vi "Bertta_v09_92.vi"() -> ()   [LabVIEW 2015]
panel:
  out "element":bool
  out "Started:":string
  in  "SHUTDOWN":bool
  in  "MASTER CONTROL":bool
  in  "Tab Control":T1(tab)
  out "Output File":path caption="selected path"
  in  "Browse folder":path=path "" caption="start path"
  in  "Read Seq":bool
  in  "Save Seq":bool
  in  "Configuration file":path=path "C:/Users/shresplab/Desktop/BerttaConfiguration.lvm" caption="Filename"
  in  "OK Button 2":bool
  out "Boolean":bool
  in  "User (initials)":string
  in  "Project name":string
  in  "Description":string
  out "PUMP1":bool
  out "Target amount":dbl
  out "Scale weight":dbl
  out "Amount now":dbl
  out "Flow rate":dbl
  out "Time to target":dbl format="%<%H:%M:%S>t"
  out "Current step":dbl
  out "Target":dbl
  out "Amount now":dbl
  out "Amount now":dbl
  out "Target":dbl
  out "Current step":dbl
  out "Time to target":dbl format="%<%H:%M:%S>t"
  out "Flow rate":dbl
  out "Amount now":dbl
  out "Scale weight":dbl
  out "Target amount":dbl
  out "PUMP2":bool
  out "Sensor OK 6":bool
  out "Sensor OK 5":bool
  out "Sensor OK 4":bool
  out "Sensor OK 3":bool
  in  "OK Button":bool
  in  "Add comment":string
  out "PUMP3":bool
  out "Target amount":dbl
  out "Scale weight":dbl
  out "Amount now":dbl
  out "Flow rate":dbl
  out "Time to target":dbl format="%<%H:%M:%S>t"
  out "Current step":dbl
  out "Target":dbl
  out "Amount now":dbl
  out "Tr":dbl
  out "Tj in":dbl
  out "Tj out":dbl
  out "T set":dbl
  out "Current step":i32
  out "RPM":dbl
  out "Torque 2":dbl
  out "Waveform Chart 5":dynamicdata(graph)
  out "Waveform Chart 6":dynamicdata(graph)
  out "Waveform Chart 7":dynamicdata(graph)
  in  "Tab Control 2":T2(tab)
  out "Waveform Chart 3":dynamicdata(graph)
  out "Waveform Chart 8":dynamicdata(graph)
  out "Waveform Chart 11":dynamicdata(graph)
  out "Waveform Chart 13":dynamicdata(graph)
  out "Waveform Chart 9":dynamicdata(graph)
  out "Table":string[][](table)=[["14.8.2017 18.06.59", "0,000000", "417,670000", "-0,150000", "1,000000", "22,220000", "23,366837", "23,574959", "23,985852", "23,690000", "240,000000", "4,000000", "0,000000", "397,000000", "-397,000000", "1,000000"], ["14.8.2017 18.07.06", "0,000000", "417,640000", "-0,120000", "1,000000", "22,220000", "23,763115", "23,906257", "23,985694", "23,680000", "240,000000", "4,000000", "0,000000", "397,000000", "-397,000000", "1,000000"], ["14.8.2017 18.07.13", "0,000000", "417,640000", "-0,120000", "1,000000", "22,220000", "23,965922", "24,013440", "23,984906", "23,670000", "240,000000", "4,100000", "3,000000", "397,000000", "-397,000000", "1,000000"], ["14.8.2017 18.07.21", "0,000000", "417,640000", "-0,120000", "1,000000", "22,220000", "23,943860", "23,900110", "23,987113", "23,670000", "240,000000", "4,000000", "0,000000", "397,000000", "-397,000000", "1,000000"], ["14.8.2017 18.07.28", "0,000000", "417,640000", "-0,120000", "1,000000", "22,220000", "23,736328", "23,600018", "23,989004", "23,660000", "240,000000", "4,000000", "0,000000", "397,000000", "-397,000000", "1,000000"], ["14.8.2017 18.07.36", "0,000000", "417,640000", "-0,120000", "1,000000", "22,220000", "23,480910", "23,324538", "23,991053", "23,660000", "240,000000", "4,000000", "0,000000", "397,000000", "-397,000000", "1,000000"], ["14.8.2017 18.07.43", "0,000000", "417,640000", "-0,120000", "2,000000", "22,220000", "23,195579", "23,008270", "23,999093", "23,650000", "240,000000", "4,000000", "0,000000", "397,000000", "-397,000000", "1,000000"], ["14.8.2017 18.07.51", "0,000000", "417,650000", "-417,650000", "1,000000", "22,220000", "22,862541", "22,649021", "24,003979", "23,650000", "240,000000", "4,000000", "0,000000", "397,000000", "-397,000000", "2,000000"], ["14.8.2017 18.07.58", "0,000000", "417,640000", "0,010000", "1,000000", "22,220000", "22,541353", "22,354878", "24,005398", "23,650000", "240,000000", "4,000000", "0,000000", "397,000000", "-397,000000", "1,000000"], ["14.8.2017 18.08.06", "0,000000", "417,640000", "0,010000", "1,000000", "22,220000", "22,347931", "22,253738", "24,007605", "23,640000", "240,000000", "4,100000", "0,000000", "397,000000", "-397,000000", "1,000000"], ["14.8.2017 18.08.13", "0,000000", "417,640000", "0,010000", "1,000000", "22,220000", "22,329030", "22,302102", "24,006028", "23,640000", "240,000000", "4,000000", "0,000000", "395,820000", "-395,820000", "1,000000"], ["14.8.2017 18.08.20", "0,000000", "417,640000", "0,010000", "1,000000", "22,220000", "22,466849", "22,511320", "24,002403", "23,630000", "240,000000", "4,000000", "0,000000", "395,830000", "-0,010000", "1,000000"], ["14.8.2017 18.08.28", "0,000000", "417,640000", "0,010000", "1,000000", "22,220000", "22,707062", "22,835101", "24,000984", "23,620000", "240,000000", "4,000000", "0,000000", "395,830000", "-0,010000", "1,000000"], ["14.8.2017 18.08.35", "0,000000", "417,640000", "0,010000", "1,000000", "22,220000", "23,054104", "23,232979", "24,001299", "23,600000", "240,000000", "4,000000", "0,000000", "395,830000", "-0,010000", "1,000000"], ["14.8.2017 18.08.43", "0,000000", "417,640000", "0,010000", "1,000000", "22,220000", "23,412371", "23,522793", "24,002560", "23,590000", "240,000000", "4,000000", "0,000000", "395,820000", "0,000000", "1,000000"], ["14.8.2017 18.08.51", "0,000000", "417,640000", "0,010000", "1,000000", "22,220000", "23,596247", "23,656125", "24,003821", "23,580000", "240,000000", "4,000000", "0,000000", "395,820000", "0,000000", "1,000000"]]
  in  "?":bool
  in  "Time":dbl format="Time to target (min):                %#_g"
  out "Current temp":dbl format="Current temperature (S1):   %#_6g"
  in  "OK Button 3":bool
  in  "T ext / T ext 2":enum32{"Sensor 1", "Sensor 2"}(radio)
  out "Sensor OK":bool
  in  "T fail":dbl=20.0 format="Failsafe temperature:              %#_g"
  in  "Setpoint":dbl=20.0 format="Temperature target:                %#_6g"
  in  "Manual select":T3(radio)
  out "Waveform Chart":dynamicdata(graph)
  out "T external 2":dbl format="Current temperature (S2):    %#_g"
  in  "UPDATE TEMP":bool
  out "Led11 5":bool
  out "RPM":dbl format="%_4f"
  out "Led10 3":bool
  out "Led9 3":bool
  out "Led8 3":bool
  out "Led7 3":bool
  out "Led6 3":bool
  out "Led5 3":bool
  out "Led4 3":bool
  out "Led3 3":bool
  out "Led2 3":bool
  out "Led1 3":bool
  in  "PumpSeq 4":dbl[][](array[numeric])=[[1.0, 1.0, 0.0, 0.0, 0.0, 0.0, 0.0, 0.0, 0.0, 0.0], [2.0, 1.0, 0.0, 0.0, 0.0, 0.0, 0.0, 0.0, 0.0, 0.0], [3.0, 1.0, 0.0, 0.0, 0.0, 0.0, 0.0, 0.0, 0.0, 0.0], [0.0, 0.0, 0.0, 0.0, 0.0, 0.0, 0.0, 0.0, 0.0, 0.0], [0.0, 0.0, 0.0, 0.0, 0.0, 0.0, 0.0, 0.0, 0.0, 0.0], [0.0, 0.0, 0.0, 0.0, 0.0, 0.0, 0.0, 0.0, 0.0, 0.0], [0.0, 0.0, 0.0, 0.0, 0.0, 0.0, 0.0, 0.0, 0.0, 0.0], [0.0, 0.0, 0.0, 0.0, 0.0, 0.0, 0.0, 0.0, 0.0, 0.0], [0.0, 0.0, 0.0, 0.0, 0.0, 0.0, 0.0, 0.0, 0.0, 0.0], [0.0, 0.0, 0.0, 0.0, 0.0, 0.0, 0.0, 0.0, 0.0, 0.0]]
  in  "?":bool
  out "Flow rate (g/min)":dbl
  out "Scale reading":dbl
  out "Step amount now":dbl
  in  "Grams / min":dbl
  out "Waveform Chart 14":dynamicdata(graph)
  in  "?":bool
  out "Total amount now":dbl
  out "Led11 4":bool
  in  "Reset 5":bool
  out "Elapsed / step":i32
  out "Time to target":dbl format="%<%H:%M:%S>t"
  in  "OK Button 4":bool
  out "Led11":bool
  out "RPM":dbl format="%_4f"
  out "Led10":bool
  out "Led9":bool
  out "Led8":bool
  out "Led7":bool
  out "Led6":bool
  out "Led5":bool
  out "Led4":bool
  out "Led3":bool
  out "Led2":bool
  out "Led1":bool
  in  "PumpSeq 2":dbl[][](array[numeric])=[[1.0, 2.0, 0.0, 0.0, 0.0, 0.0, 0.0, 0.0, 0.0, 0.0], [2.0, 2.0, 0.0, 0.0, 0.0, 0.0, 0.0, 0.0, 0.0, 0.0], [3.0, 2.0, 0.0, 0.0, 0.0, 0.0, 0.0, 0.0, 0.0, 0.0], [0.0, 0.0, 0.0, 0.0, 0.0, 0.0, 0.0, 0.0, 0.0, 0.0], [0.0, 0.0, 0.0, 0.0, 0.0, 0.0, 0.0, 0.0, 0.0, 0.0], [0.0, 0.0, 0.0, 0.0, 0.0, 0.0, 0.0, 0.0, 0.0, 0.0], [0.0, 0.0, 0.0, 0.0, 0.0, 0.0, 0.0, 0.0, 0.0, 0.0], [0.0, 0.0, 0.0, 0.0, 0.0, 0.0, 0.0, 0.0, 0.0, 0.0], [0.0, 0.0, 0.0, 0.0, 0.0, 0.0, 0.0, 0.0, 0.0, 0.0], [0.0, 0.0, 0.0, 0.0, 0.0, 0.0, 0.0, 0.0, 0.0, 0.0]]
  in  "?":bool
  out "Flow rate (g/min)":dbl
  out "Scale reading":dbl
  out "Step amount now":dbl
  in  "Grams / min":dbl
  out "Waveform Chart 10":dynamicdata(graph)
  in  "?":bool
  out "Total amount now":dbl
  out "Led11":bool
  in  "Reset 3":bool
  out "Elapsed / step":i32
  out "Time to target":dbl format="%<%H:%M:%S>t"
  in  "OK Button 5":bool
  out "Led11 3":bool
  out "RPM":dbl format="%_4f"
  out "Led10 2":bool
  out "Led9 2":bool
  out "Led8 2":bool
  out "Led7 2":bool
  out "Led6 2":bool
  out "Led5 2":bool
  out "Led4 2":bool
  out "Led3 2":bool
  out "Led2 2":bool
  out "Led1 2":bool
  in  "PumpSeq 3":dbl[][](array[numeric])=[[1.0, 3.0, 0.0, 0.0, 0.0, 0.0, 0.0, 0.0, 0.0, 0.0], [2.0, 3.0, 0.0, 0.0, 0.0, 0.0, 0.0, 0.0, 0.0, 0.0], [3.0, 3.0, 0.0, 0.0, 0.0, 0.0, 0.0, 0.0, 0.0, 0.0], [0.0, 0.0, 0.0, 0.0, 0.0, 0.0, 0.0, 0.0, 0.0, 0.0], [0.0, 0.0, 0.0, 0.0, 0.0, 0.0, 0.0, 0.0, 0.0, 0.0], [0.0, 0.0, 0.0, 0.0, 0.0, 0.0, 0.0, 0.0, 0.0, 0.0], [0.0, 0.0, 0.0, 0.0, 0.0, 0.0, 0.0, 0.0, 0.0, 0.0], [0.0, 0.0, 0.0, 0.0, 0.0, 0.0, 0.0, 0.0, 0.0, 0.0], [0.0, 0.0, 0.0, 0.0, 0.0, 0.0, 0.0, 0.0, 0.0, 0.0], [0.0, 0.0, 0.0, 0.0, 0.0, 0.0, 0.0, 0.0, 0.0, 0.0]]
  in  "?":bool
  out "Flow rate (g/min)":dbl
  out "Scale reading":dbl
  out "Step amount now":dbl
  in  "Grams / min":dbl
  out "Waveform Chart 12":dynamicdata(graph)
  in  "?":bool
  out "Total amount now":dbl
  out "Led11 2":bool
  in  "Reset 4":bool
  out "Elapsed / step":i32
  out "Time to target":dbl format="%<%H:%M:%S>t"
  in  "OK Button 6":bool
  in  "Bypass select 2":enum32{"Remote", "Manual"}(radio)=enum."Manual"
  in  "Port":dbl=13.0
  out "RPM":dbl
  out "Torque":dbl
  in  "Set RPM":dbl(slide) scale=0.0..2000.0
  out "Waveform Chart 4":dynamicdata(graph)
  in  "OK Button 7":bool
  out "output array":dbl[](array[numeric])
  in  "dev1":i32=1
  in  "dev2":i32=2
  in  "dev3":i32=3
  in  "dev4":i32=4
  in  "dev5":i32=5
  in  "dev6":i32=5
  in  "dev8":i32
  in  "port1":i32=9
  in  "port2":i32=9
  in  "port3":i32=13
  in  "port4":i32=13
  in  "port5":i32=10
  in  "port6":i32=11
  in  "port7":i32=12
  in  "port8":i32
  in  "dev7":i32=5
  in  "Treshold (T/C)":dbl=0.5
  out "DAQ 9217 (PT100)":errorcluster
  out "Config File":dbl[][](array[numeric])
  # "Temperature sensor:"
  # "Manual control:"
  # "PUMP & SCALE 1"
  # "STEP"
  # "TOTAL"
  # "PUMP & SCALE 2"
  # "STEP"
  # "TOTAL"
  # "PUMP & SCALE 3"
  # "STEP"
  # "TOTAL"
  # "Temperature control parameter"
  # "Secondary temperature sensor"
  # "Grams    /   min"
  # "End of sequence"
  # "Manual control"
  # "Grams    /   min"
  # "End of sequence"
  # "Manual control"
  # "Grams    /   min"
  # "End of sequence"
  # "Manual control"
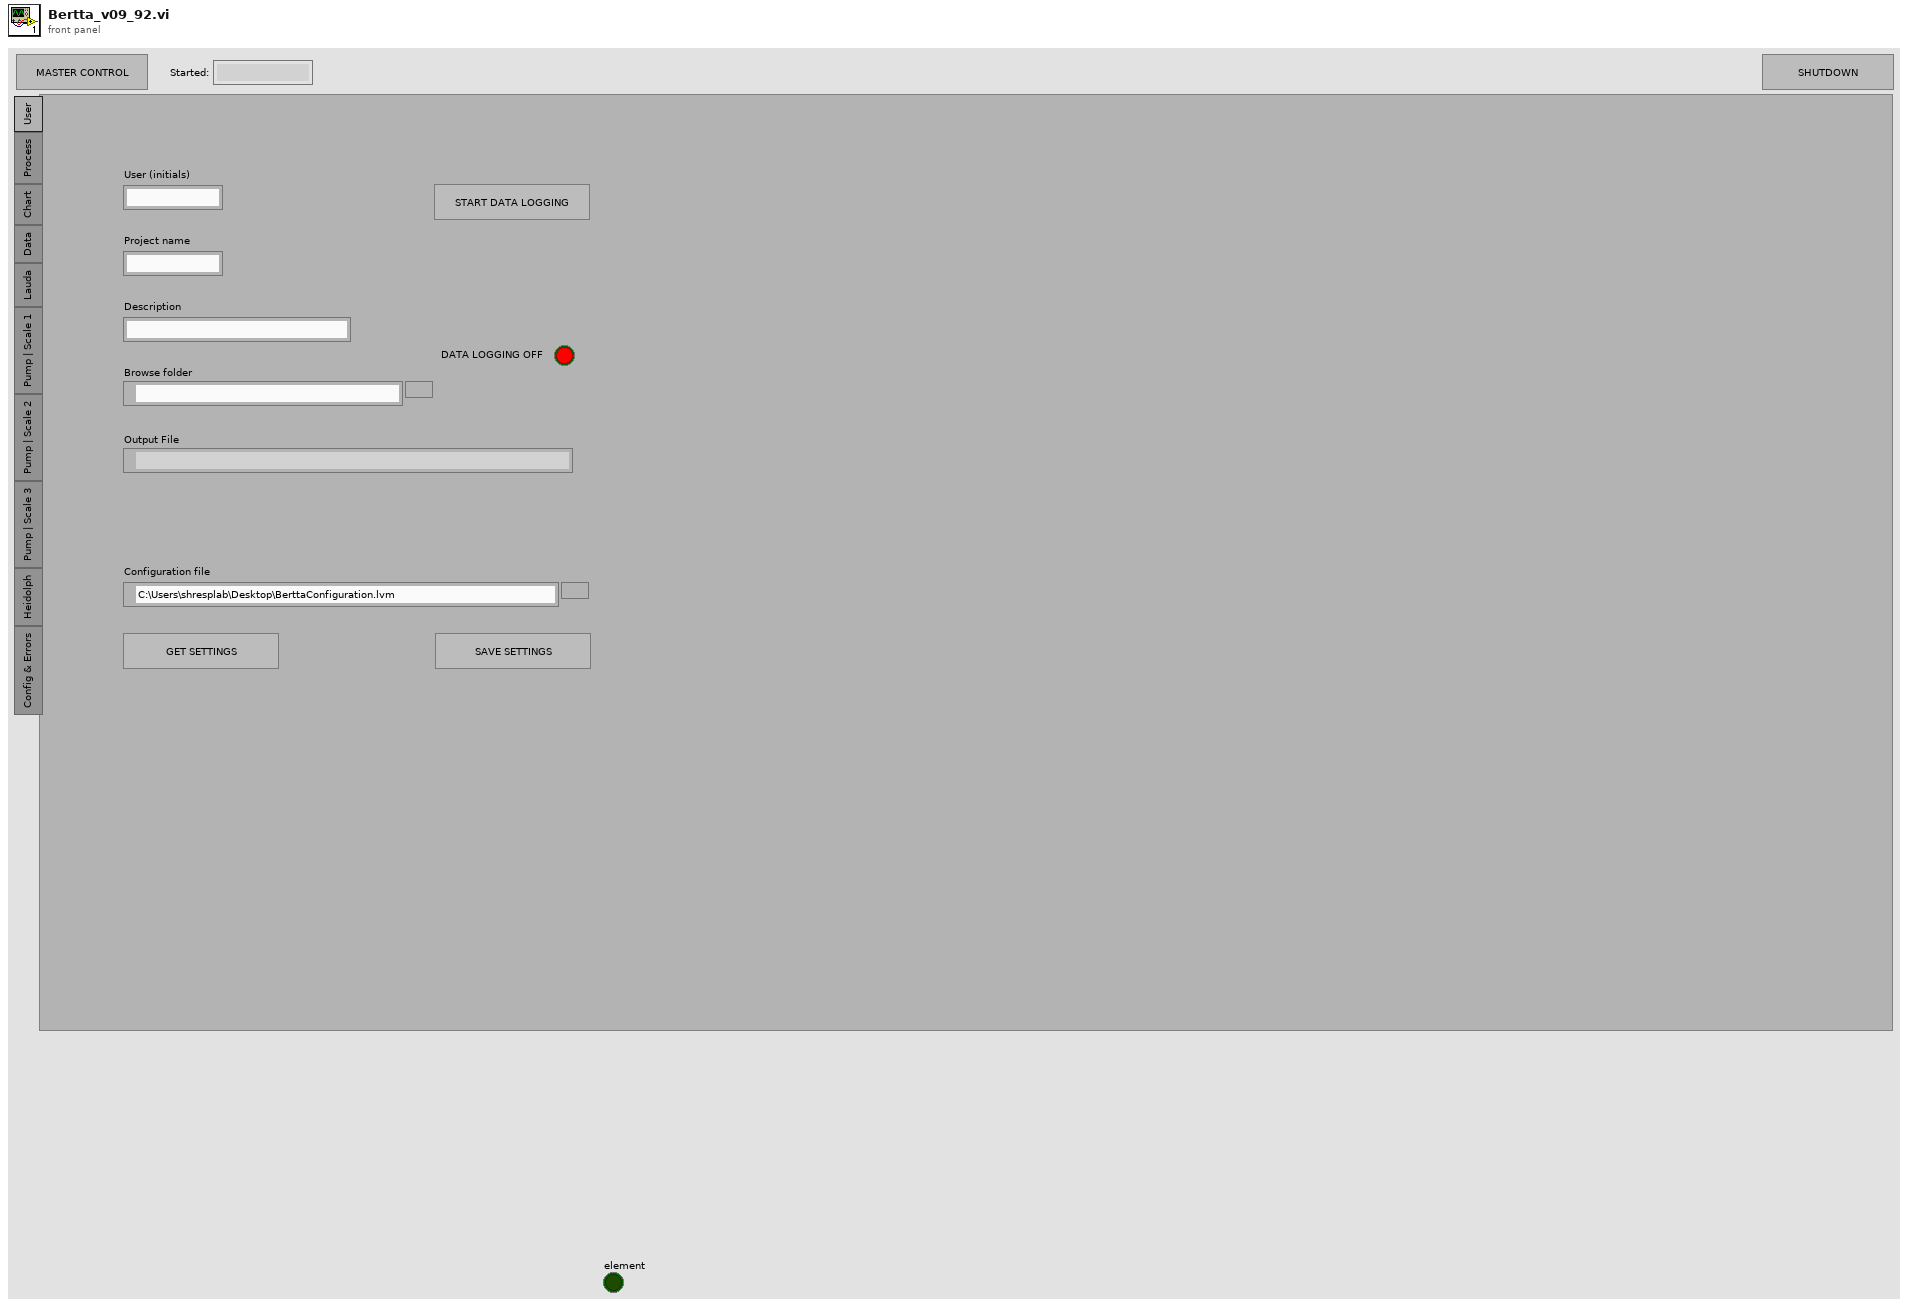
[diagram p1: front panel]
types:
  T1 = enum32{"User", "Process", "Chart", "Data", "Lauda", "Pump | Scale 1", "Pump | Scale 2", "Pump | Scale 3", "Heidolph", "Config & Errors"}
  T2 = enum32{"Temperatures", "Scale / Pump 1", "Scale / Pump 2", "Scale / Pump 3", "RPM / torque"}
  T3 = enum32{"Reactor temperature", "Jacket temperature"}
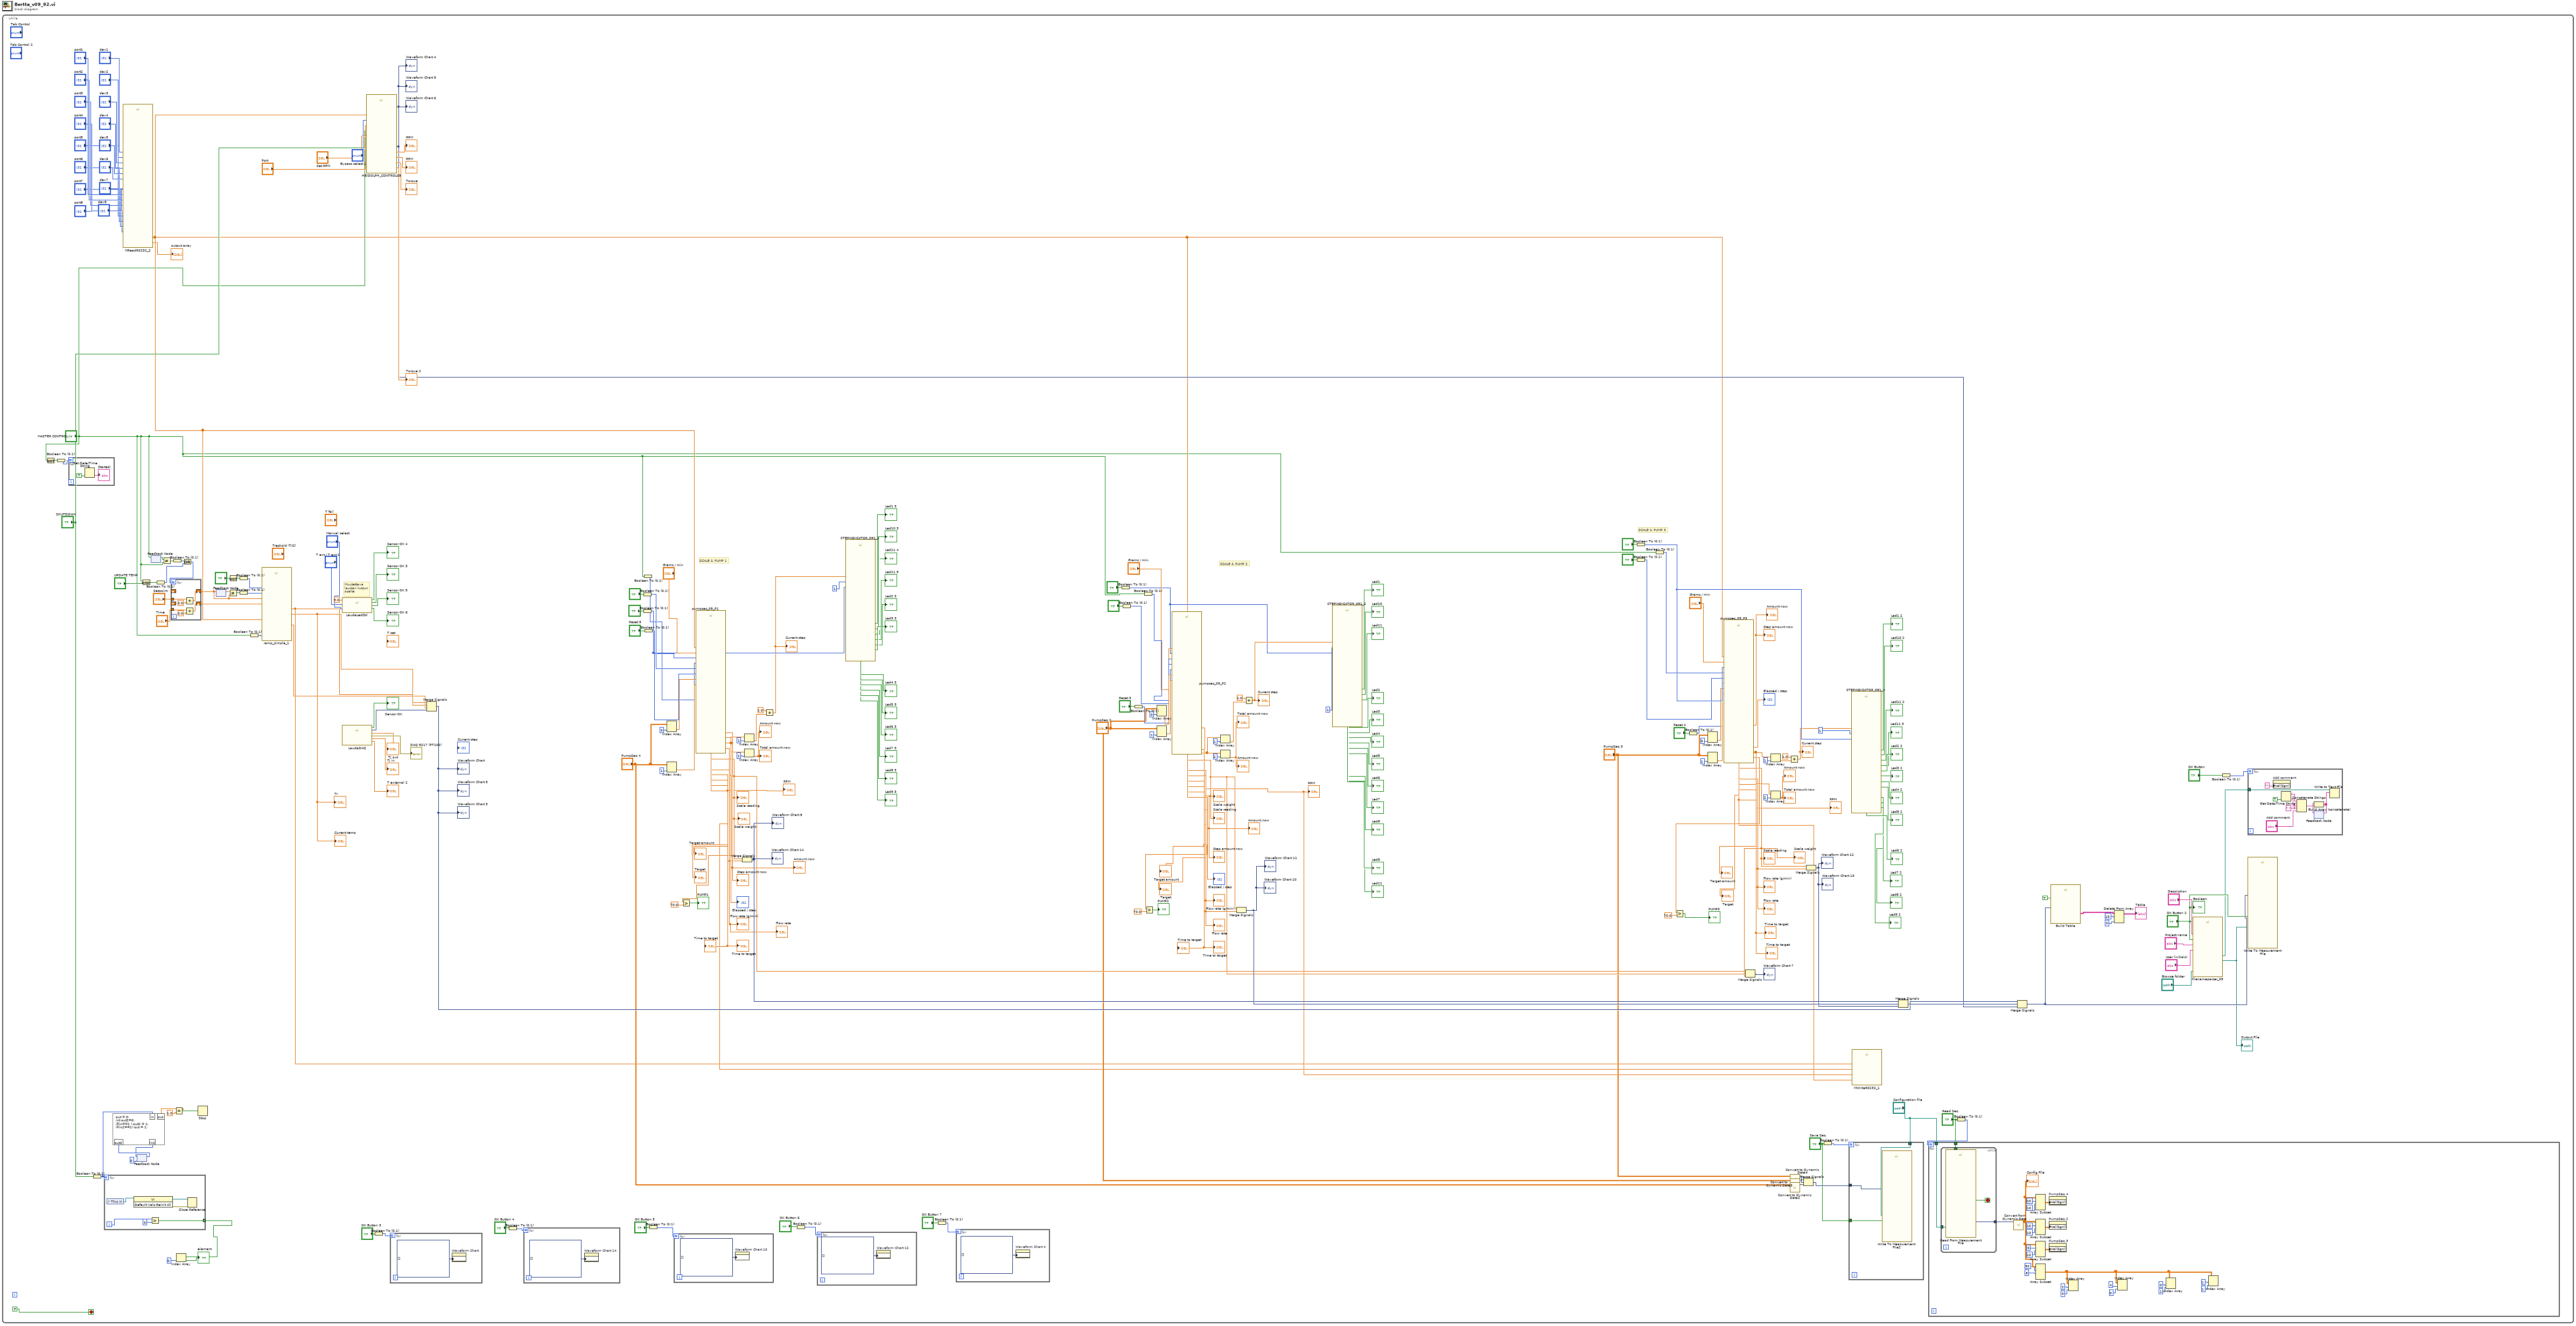
[diagram p0: block diagram]
diagram:
  n1 = while {
    stop <- FALSE stop-if-true
    # "Muutettava\nlaudan kutsun \nosalta"
    # "SCALE & PUMP 1"
    # "SCALE & PUMP 3"
    # "SCALE & PUMP 2"
    n2 = Not(x="MASTER CONTROL") -> (.not. x?=w236:bool)
    n3 = Boolean To (0,1)(Boolean=w236) -> (0, 1=w237:i16)
    n4 = for {
      N: w237 -> [_]
      n5 = Get Date/Time String(want seconds? (F)=TRUE) -> (time string=→"Started:":string)  [unwired: 2 in, 1 out]
    }
    n6 = Boolean To (0,1)(Boolean="SHUTDOWN") -> (0, 1=w219:i16)
    n7 = for {
      N: w219 -> [_]
      tunnel: [w300] -> w235 mode=indexing
      i -> [w302]
      n8 = control-ref of="This VI"() -> (w305:refnum<vi>)
      n9 = invoke class="VI" method="Default Vals.Reinit All"(reference=w305) -> (reference out=w303:refnum<vi>, error out=w304:errorcluster)  [unwired: 2 in, 1 out]
      n10 = Greater?(x=w302, y=0) -> (0:w300:bool)
      n11 = Close Reference(reference=w303, error in (no error)=w304) -> ()  [unwired: 1 out]
    }
    n12 = call "MReadRS232_2.vi"("port1"="port1", "dev1"="dev1", "port2"="port2", "dev2"="dev2", "port3"="port3", "dev7"="dev7", "dev8"="dev8", "port7"="port7", "port8"="port8", "dev5"="dev5", "port5"="port5", "dev4"="dev4", "dev6"="dev6", "port6"="port6", "port4"="port4", "dev3"="dev3") -> ("output array"=→"output array":dbl[], "params"=w40:dbl[])  [unwired: 2 in]
    n13 = feedback #1(0) -> (w217:i32)
    n14 = formula code="out = 0;\nint out2=0;\nif(in==1 ) out2 = 1;\nif(in2==1) out = 1;"("in"=w219, "in2"=w217) -> ("out"=w221:dbl, "out2"=w218:i32)
    n15 = feedback-in #1(w218) -> ()
    n16 = And(x="MASTER CONTROL", y="UPDATE TEMP") -> (x .and. y?=w32:bool)
    n17 = feedback #2() -> (w23:bool)  [unwired: 1 in]
    n18 = feedback-in #2("MASTER CONTROL") -> ()
    n19 = Boolean To (0,1)(Boolean=w32) -> (0, 1=w20:i16)
    n20 = Not Equal?(x=w23, y="MASTER CONTROL") -> (x != y?=w22:bool)
    n21 = Boolean To (0,1)(Boolean=w22) -> (0, 1=w19:i16)
    n22 = Equal?(x=w221, y=1.0) -> (x = y?=w220:bool)
    n23 = Index Array(array=w235, index=0) -> (element=→"element":bool)
    n24 = Or(x=w19, y=w20) -> (x .or. y?=w18:i16)
    n25 = for {
      N: w18 -> [_]
      tunnel: "Time" -> [w252]
      shift-right: [w251] -> w34
      shift-left: _ -> [_]
      tunnel: "Setpoint" -> [w249]
      shift-right: [w248] -> w30
      shift-left: _ -> [_]
      n26 = Add(x=w249, y=0.0) -> (x+y=w248:dbl)
      n27 = Add(x=w252, y=0.0) -> (x+y=w251:dbl)
    }
    n28 = Stop(stop? (T)=w220) -> ()
    n29 = feedback-in #3(w30) -> ()
    n30 = feedback #3() -> (w31:dbl)  [unwired: 1 in]
    n31 = Not(x="?") -> (.not. x?=w26:bool)
    n32 = Not Equal?(x=w31, y=w30) -> (x != y?=w29:bool)
    n33 = Boolean To (0,1)(Boolean=w26) -> (0, 1=w28:i16)
    n34 = Boolean To (0,1)(Boolean=w29) -> (0, 1=w24:i16)
    n35 = Boolean To (0,1)(Boolean="MASTER CONTROL") -> (0, 1=w25:i16)
    n36 = call "ramp_simple_1.vi"("array"=w40, "time_set"=w34, "T_sp"=w30, "master"=w25, "reset"=w24, "pause"=w28) -> ("T control"=w39:dbl, "Tr"=w38:dbl, "Tin"=w37:dbl)  [unwired: 2 in, 1 out]
    "Tr" <- w38
    "Current temp" <- w38
    n37 = call "LaudaLedCtrl.vi"("Manual select"="Manual select", "T ext / T ext in"="T ext / T ext 2", "Lauda port"=9.0) -> ("Sensor OK 5"=→"Sensor OK 5":bool, "Sensor OK 3"=→"Sensor OK 3":bool, "Sensor OK 4"=→"Sensor OK 4":bool, "Sensor OK 6"=→"Sensor OK 6":bool)  [unwired: 5 in]
    n38 = call "LaudaDAQ.vi"() -> ("error out"=→"DAQ 9217 (PT100)":errorcluster, 1:"Tj out"=→"Tj out":dbl, "data"=w108:dynamicdata, "Sensor OK"=→"Sensor OK":bool, 4:"Tj out"=→"Tj in":dbl, "T external 2"=→"T external 2":dbl)  [unwired: 6 in]
    n39 = call "HEIDOLPH_CONTROL09.vi"("master"="MASTER CONTROL", "Array"=w40, "shutdown"="SHUTDOWN", "Bypass select"="Bypass select 2", "Set RPM"="Set RPM", "Device port"="Port") -> ("Dynamic Data"=w109:dynamicdata, "RPM"=→"RPM":dbl, "RPM 2"=→"RPM":dbl, "Torque"=→"Torque":dbl, "Torque 2"=→"Torque 2":dbl)  [unwired: 1 in]
    "Waveform Chart 4" <- w109
    "Waveform Chart 6" <- w109
    "Waveform Chart 9" <- w109
    n40 = Boolean To (0,1)(Boolean="OK Button 3") -> (0, 1=w51:i16)
    n41 = for {
      N: w51 -> [_]
      n42 = property on="Waveform Chart" class="WFChart (strict)"("History Data"=dynamicdata[] []) -> ()  [unwired: 2 in, 2 out]
    }
    n43 = Merge Signals(w39, w38, w37, w108) -> (w110:dynamicdata)
    "Waveform Chart 3" <- w110
    "Waveform Chart" <- w110
    "Waveform Chart 5" <- w110
    n44 = Boolean To (0,1)(Boolean="OK Button 4") -> (0, 1=w49:i16)
    n45 = for {
      N: w49 -> [_]
      n46 = property on="Waveform Chart 14" class="WFChart (strict)"("History Data"=dynamicdata[] []) -> ()  [unwired: 2 in, 2 out]
    }
    n47 = Boolean To (0,1)(Boolean="?") -> (0, 1=w118:i16)
    n48 = Boolean To (0,1)(Boolean="?") -> (0, 1=w122:i16)
    n49 = Boolean To (0,1)(Boolean="MASTER CONTROL") -> (0, 1=w114:i16)
    n50 = Boolean To (0,1)(Boolean="Reset 5") -> (0, 1=w121:i16)
    n51 = Boolean To (0,1)(Boolean="OK Button 5") -> (0, 1=w47:i16)
    n52 = Index Array(array="PumpSeq 4", index (col)=0) -> (element=w126:dbl[])  [unwired: 1 in]
    n53 = Index Array(array="PumpSeq 4", index (col)=1) -> (element=w147:dbl[])  [unwired: 1 in]
    n54 = for {
      N: w47 -> [_]
      n55 = property on="Waveform Chart 10" class="WFChart (strict)"("History Data"=dynamicdata[] []) -> ()  [unwired: 2 in, 2 out]
    }
    n56 = call "pumpsec_09_P1.vi"("reset"=w121, "master"=w114, "manual"=w118, "pause"=w122, "Array"=w40, "Target"=w126, "fr_manual"="Grams / min", "Time"=w147) -> ("pumpCtrl"=w92:dbl, "totaltarget"=→"Target":dbl, "target_step"=→"Target amount":dbl, "REGLO D"=w58:dbl, "time_to_target"=→"Time to target" →"Time to target":dbl, "step_fr"=w69:dbl, "amount_step"=→"Amount now" →"Step amount now":dbl, "Scale"=w104:dbl, "elapsed_step"=→"Elapsed / step":dbl, "params"=w144:dbl[])  [unwired: 8 in, 2 out]
    "Flow rate" <- w69
    "Scale weight" <- w104
    "Scale reading" <- w104
    "Flow rate (g/min)" <- w69
    "RPM" <- w58
    n57 = Greater?(x=w92, y=70.0) -> (0:→"PUMP1":bool)
    n58 = Merge Signals(w104, w69) -> (w113:dynamicdata)
    "Waveform Chart 8" <- w113
    "Waveform Chart 14" <- w113
    n59 = Index Array(array=w144, index=1) -> (element=w141:dbl)
    n60 = Index Array(array=w144, index=2) -> (element=→"Amount now" →"Total amount now":dbl)
    n61 = Add(x=1.0, y=w141) -> (x+y=w70:dbl)
    "Current step" <- w70
    n62 = Boolean To (0,1)(Boolean="OK Button 6") -> (0, 1=w45:i16)
    n63 = for {
      N: w45 -> [_]
      n64 = property on="Waveform Chart 12" class="WFChart (strict)"("History Data"=dynamicdata[] []) -> ()  [unwired: 2 in, 2 out]
    }
    n65 = call "STEPINDICATOR_091_2.vi"("current step"=w70, "enable"=i16 1, "manual"=w118) -> ("Led 8"=→"Led8 3":bool, "Led 10"=→"Led10 3":bool, "Led 11"=→"Led11 4":bool, "Led 7"=→"Led7 3":bool, "Led 1"=→"Led1 3":bool, "Led 6"=→"Led6 3":bool, "Led 2"=→"Led2 3":bool, "Led 12"=→"Led11 5":bool, "Led 5"=→"Led5 3":bool, "Led 4"=→"Led4 3":bool, "Led 3"=→"Led3 3":bool, "Led 9"=→"Led9 3":bool)  [unwired: 1 in]
    n66 = Boolean To (0,1)(Boolean="OK Button 7") -> (0, 1=w43:i16)
    n67 = for {
      N: w43 -> [_]
      n68 = property on="Waveform Chart 4" class="WFChart (strict)"("History Data"=dynamicdata[] []) -> ()  [unwired: 2 in, 2 out]
    }
    n69 = Boolean To (0,1)(Boolean="?") -> (0, 1=w181:i16)
    n70 = Boolean To (0,1)(Boolean="?") -> (0, 1=w208:i16)
    n71 = Boolean To (0,1)(Boolean="Reset 3") -> (0, 1=w206:i16)
    n72 = Boolean To (0,1)(Boolean="MASTER CONTROL") -> (0, 1=w200:i16)
    n73 = Index Array(array="PumpSeq 2", index (col)=0 ("disabled index (col)")) -> (element=w211:dbl[])  [unwired: 1 in]
    n74 = Index Array(array="PumpSeq 2", index (col)=1 ("disabled index (col)")) -> (element=w210:dbl[])  [unwired: 1 in]
    n75 = call "pumpsec_09_P2.vi"("reset"=w206, "master"=w200, "manual"=w181, "pause"=w208, "Array"=w40, "Target"=w211, "fr_manual"="Grams / min", "Time"=w210) -> ("pumpCtrl"=w88:dbl, "totaltarget"=→"Target":dbl, "target_step"=→"Target amount":dbl, "REGLO D"=w57:dbl, "time_to_target"=→"Time to target" →"Time to target":dbl, "step_fr"=w107:dbl, "amount_step"=→"Amount now" →"Step amount now":dbl, "Scale"=w103:dbl, "elapsed_step"=→"Elapsed / step":dbl, "params"=w201:dbl[])  [unwired: 8 in, 2 out]
    "Scale weight" <- w103
    "Flow rate" <- w107
    "Scale reading" <- w103
    "Flow rate (g/min)" <- w107
    "RPM" <- w57
    n76 = Greater?(x=w88, y=70.0) -> (0:→"PUMP2":bool)
    n77 = Index Array(array=w201, index=1) -> (element=w204:dbl)
    n78 = Index Array(array=w201, index=2) -> (element=→"Amount now" →"Total amount now":dbl)
    n79 = Merge Signals(w103, w107) -> (w115:dynamicdata)
    "Waveform Chart 11" <- w115
    "Waveform Chart 10" <- w115
    n80 = Add(x=1.0, y=w204) -> (x+y=w198:dbl)
    "Current step" <- w198
    n81 = call "STEPINDICATOR_091_2.vi"("current step"=w198, "enable"=i16 1, "manual"=w181) -> ("Led 8"=→"Led8":bool, "Led 10"=→"Led10":bool, "Led 11"=→"Led11":bool, "Led 7"=→"Led7":bool, "Led 1"=→"Led1":bool, "Led 6"=→"Led6":bool, "Led 2"=→"Led2":bool, "Led 12"=→"Led11":bool, "Led 5"=→"Led5":bool, "Led 4"=→"Led4":bool, "Led 3"=→"Led3":bool, "Led 9"=→"Led9":bool)  [unwired: 1 in]
    n82 = Boolean To (0,1)(Boolean="?") -> (0, 1=w175:i16)
    n83 = Boolean To (0,1)(Boolean="?") -> (0, 1=w174:i16)
    n84 = Boolean To (0,1)(Boolean="MASTER CONTROL") -> (0, 1=w176:i16)
    n85 = Boolean To (0,1)(Boolean="Reset 4") -> (0, 1=w156:i16)
    n86 = Index Array(array="PumpSeq 3", index (col)=0 ("disabled index (col)")) -> (element=w159:dbl[])  [unwired: 1 in]
    n87 = Index Array(array="PumpSeq 3", index (col)=1 ("disabled index (col)")) -> (element=w158:dbl[])  [unwired: 1 in]
    n88 = call "pumpsec_09_P3.vi"("reset"=w156, "master"=w176, "manual"=w175, "pause"=w174, "Array"=w40, "Target"=w159, "fr_manual"="Grams / min", "Time"=w158) -> ("pumpCtrl"=w85:dbl, "totaltarget"=→"Target":dbl, "target_step"=→"Target amount":dbl, "REGLO D"=w56:dbl, "time_to_target"=→"Time to target" →"Time to target":dbl, "step_fr"=w106:dbl, "amount_step"=→"Amount now" →"Step amount now":dbl, "Scale"=w102:dbl, "elapsed_step"=→"Elapsed / step":dbl, "params"=w149:dbl[])  [unwired: 8 in, 2 out]
    "Scale weight" <- w102
    "Flow rate" <- w106
    "Scale reading" <- w102
    "Flow rate (g/min)" <- w106
    "RPM" <- w56
    n89 = Greater?(x=w85, y=70.0) -> (0:→"PUMP3":bool)
    n90 = Merge Signals(w104, w103, w102) -> (→"Waveform Chart 7":dynamicdata)
    n91 = Index Array(array=w149, index=1) -> (element=w150:dbl)
    n92 = Index Array(array=w149, index=2) -> (element=→"Amount now" →"Total amount now":dbl)
    n93 = Add(x=1.0, y=w150) -> (x+y=w148:dbl)
    "Current step" <- w148
    n94 = call "Convert to Dynamic Data4"("2D Array"="PumpSeq 3") -> ("Dynamic Data Type"=w61:dynamicdata)  [unwired: 3 in]
    n95 = call "Convert to Dynamic Data3"("2D Array"="PumpSeq 2") -> ("Dynamic Data Type"=w63:dynamicdata)  [unwired: 3 in]
    n96 = call "Convert to Dynamic Data2"("2D Array"="PumpSeq 4") -> ("Dynamic Data Type"=w66:dynamicdata)  [unwired: 3 in]
    n97 = Merge Signals(w61, w63, w66) -> (w65:dynamicdata)
    n98 = Merge Signals(w102, w106) -> (w112:dynamicdata)
    "Waveform Chart 13" <- w112
    "Waveform Chart 12" <- w112
    n99 = Boolean To (0,1)(Boolean="Save Seq") -> (0, 1=w60:i16)
    n100 = for {
      N: w60 -> [_]
      tunnel: w65 -> [w298]
      tunnel: "Configuration file" -> [w299]
      tunnel: "Save Seq" -> [w297]
      n101 = call "Write To Measurement File2"("Signals"=w298, "Reset"=w297, "Filename"=w299) -> ()  [unwired: 14 in, 3 out]
    }
    n102 = call "STEPINDICATOR_091_4.vi"("current step"=w148, "enable"=i16 1, "manual"=w175) -> ("Led 8"=→"Led8 2":bool, "Led 10"=→"Led10 2":bool, "Led 11"=→"Led11 2":bool, "Led 7"=→"Led7 2":bool, "Led 1"=→"Led1 2":bool, "Led 6"=→"Led6 2":bool, "Led 2"=→"Led2 2":bool, "Led 12"=→"Led11 3":bool, "Led 5"=→"Led5 2":bool, "Led 4"=→"Led4 2":bool, "Led 3"=→"Led3 2":bool, "Led 9"=→"Led9 2":bool)  [unwired: 1 in]
    n103 = call "MWriteRS232_1.vi"("P3"=w56, "P2"=w57, "P1"=w58, "LAUDA"=w39) -> ()  [unwired: 8 in]
    n104 = Merge Signals(w113, w115, w112) -> (w111:dynamicdata)
    n105 = Boolean To (0,1)(Boolean="Read Seq") -> (0, 1=w59:i16)
    n106 = for {
      N: w59 -> [_]
      tunnel: "Configuration file" -> [w270]
      tunnel: "Read Seq" -> [w269]
      n107 = while {
        tunnel: [w296] -> w292
        tunnel: w270 -> [w295]
        tunnel: w269 -> [w293]
        stop <- w294 stop-if-true
        n108 = call "Read From Measurement File"("Filename"=w295, "Reset"=w293) -> ("Signals"=w296:dynamicdata, "EOF?"=w294:bool)  [unwired: 4 in, 4 out]
      }
      n109 = call "Convert from Dynamic Data"("Dynamic Data Type"=w292) -> ("Array"=w282:dbl[][])  [unwired: 3 in]
      "Config File" <- w282
      n110 = Array Subset(array=w282, index (row)=20 ("index"), length (row)=10 ("length")) -> (w289:dbl[][])  [unwired: 2 in]
      n111 = Array Subset(array=w282, index (row)=10 ("index"), length (row)=10 ("length")) -> (w284:dbl[][])  [unwired: 2 in]
      n112 = Array Subset(array=w282, index (row)=0 ("index"), length (row)=10 ("length")) -> (w283:dbl[][])  [unwired: 2 in]
      n113 = Array Subset(array=w282, index (row)=30 ("index"), length (row)=8 ("length")) -> (w271:dbl[][])  [unwired: 2 in]
      n114 = property on="PumpSeq 4" class="Arr (strict)"("Val(Sgnl)"=w289) -> ()  [unwired: 2 in, 2 out]
      n115 = property on="PumpSeq 2" class="Arr (strict)"("Val(Sgnl)"=w284) -> ()  [unwired: 2 in, 2 out]
      n116 = property on="PumpSeq 3" class="Arr (strict)"("Val(Sgnl)"=w283) -> ()  [unwired: 2 in, 2 out]
      n117 = Index Array(array=w271, index (row)=2, index (col)=0 ("disabled index (col)")) -> ()  [unwired: 1 out]
      n118 = Index Array(array=w271, index (row)=4, index (col)=0 ("disabled index (col)")) -> ()  [unwired: 1 out]
      n119 = Index Array(array=w271, index (row)=0, index (col)=1 ("disabled index (col)")) -> ()  [unwired: 1 out]
      n120 = Index Array(array=w271, index (row)=1, index (col)=1 ("disabled index (col)")) -> ()  [unwired: 1 out]
    }
    n121 = Merge Signals(w110, w111, w109) -> (w230:dynamicdata)
    n122 = call "Build Table"("Include time data"=TRUE, "Signals"=w230) -> ("Table"=w229:string[][])  [unwired: 3 in, 6 out]
    n123 = Delete From Array(array=w229, length=13, index (col)=0 ("index (row)")) -> (array with subset deleted=→"Table":string[][])  [unwired: 1 in, 1 out]
    n124 = call "filenameparser_09.vi"("Description"="Description", "start path"="Browse folder", "Project name"="Project name", "User (initials)"="User (initials)", "OK Button in"="OK Button 2") -> ("appended path 2"=w41:path, "appended path"=w225:path)  [unwired: 4 in, 1 out]
    "Output File" <- w41
    n125 = Boolean To (0,1)(Boolean="OK Button") -> (0, 1=w224:i16)
    n126 = for {
      N: w224 -> [_]
      tunnel: w225 -> [w261]
      w265 = " " ("string")
      n127 = property on="Add comment" class="Str"("Val(Sgnl)"="" ("Value (Signaling)")) -> ()  [unwired: 2 in, 2 out]
      n128 = Get Date/Time String(want seconds? (F)=TRUE) -> (date string=w268:string, time string=w266:string)  [unwired: 2 in]
      n129 = Concatenate Strings(w268, w265, w266, w265, "Add comment") -> (w264:string)
      n130 = feedback #4() -> (w263:string[])  [unwired: 1 in]
      n131 = Build Array (concatenate)(w263, w264) -> (w262:string[])
      n132 = feedback-in #4(w262) -> ()
      n133 = Write to Text File(file (use dialog)=w261, text=w262) -> ()  [unwired: 2 in, 3 out]
    }
    n134 = call "Write To Measurement File"("Signals"=w230, "Enable"="OK Button 2", "Filename"=w41) -> ()  [unwired: 14 in, 3 out]
    "Boolean" <- "OK Button 2"
  }
